vi "extract magnetometer queue to time range.vi"(8 "error in (no error)":errorcluster, 9 "time ranges to exclude":cluster{"t0":dbl, "t1":dbl}[](array[cluster]), 10 "time range to include":cluster{"t0":dbl, "t1":dbl}={"t0"=-1.0, "t1"=-1.0}, 11 "magnetometer set queue":refnum<queue>) -> (0 "error out":errorcluster, 3 "readings in range":T1[](array[typedef]))   [LabVIEW 2017]
uses:
  typedefs/magnetomter reading set.ctl
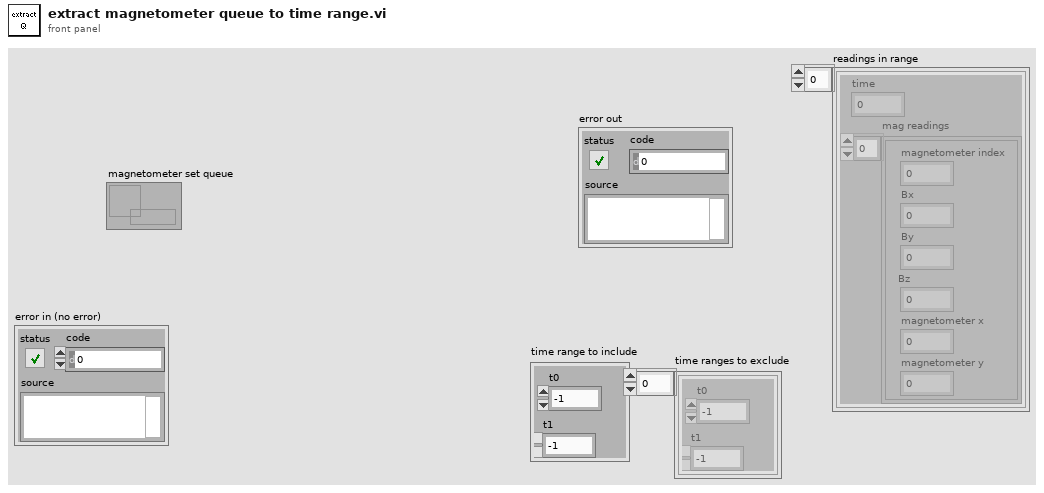
[diagram p1: front panel]
types:
  T1 = typedef "magnetomter reading set.ctl" = cluster{"time":fxp<+,48,48>, "mag readings":cluster{"magnetometer index":dbl, "Bx":dbl, "By":dbl, "Bz":dbl, "magnetometer x":dbl, "magnetometer y":dbl}[]}
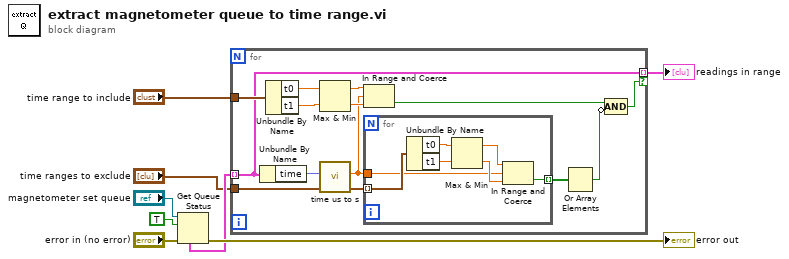
[diagram p0: block diagram]
diagram:
  n1 = Get Queue Status(queue="magnetometer set queue", return elements? (F)=TRUE, error in (no error)="error in (no error)") -> (error out=→"error out":errorcluster, elements=w4:T1[])  [unwired: 6 out]
  n2 = for {
    tunnel: w4 -> [w13] mode=indexing
    tunnel: "time range to include" -> [w21]
    tunnel: "time ranges to exclude" -> [w16]
    tunnel: [w13] -> w1 mode=indexing if=w12
    n3 = Unbundle By Name(w13) -> ("time"=w10:fxp<+,48,48>)
    n4 = Unbundle By Name(w21) -> ("t0"=w20:dbl, "t1"=w19:dbl)
    n5 = Max & Min(x=w20, y=w19) -> (max(x,y)=w18:dbl, min(x,y)=w17:dbl)
    n6 = call "time us to s.vi"("time (us)"=w10) -> ("time (s)"=w11:dbl)  [unwired: 10 in]
    n7 = In Range and Coerce(upper limit=w18, x=w11, lower limit=w17) -> (In Range?=w14:bool)  [unwired: 1 out]
    n8 = for {
      tunnel: w16 -> [w24] mode=indexing
      tunnel: [w23] -> w15 mode=indexing
      tunnel: w11 -> [w22]
      n9 = Unbundle By Name(w24) -> ("t0"=w28:dbl, "t1"=w27:dbl)
      n10 = Max & Min(x=w28, y=w27) -> (max(x,y)=w26:dbl, min(x,y)=w25:dbl)
      n11 = In Range and Coerce(upper limit=w26, x=w22, lower limit=w25) -> (In Range?=w23:bool)  [unwired: 1 out]
    }
    n12 = Or Array Elements(Boolean array=w15) -> (logical OR=w9:bool)
    n13 = Compound Arithmetic op=AND(w14, invert w9) -> (w12:bool)
  }
  "readings in range" <- w1
